vi "CHS_TRAJECTORY_EXECUTE_REL.vi"(6 "Pass_Through_Time":dbl=-1.0 format="%33.4f", 8 "Init":bool, 11 "TrajectoryName":string) -> (1 "Complete":bool, 2 "AtReference":bool, 3 "Chassis Velocity Target SI":T1 {"vOmega" format="%10.3f"; "vY" format="%10.3f"; "vX" format="%10.3f"})   [LabVIEW 2019]
uses:
  CHS_TRAJECTORY_GLOBALS.vi
  <vilib>/Rock Robotics/WPI/ThirdParty/JAS_Junk/TrajLib/Trajectory_Library.lvlib
  <vilib>/Rock Robotics/WPI/ThirdParty/ChoreoLib/ChoreoLib.lvlib
  <vilib>/Rock Robotics/WPI/ThirdParty/JAS_Junk/TrajLib/TypeDef/CHASSIS_SPEEDS.ctl
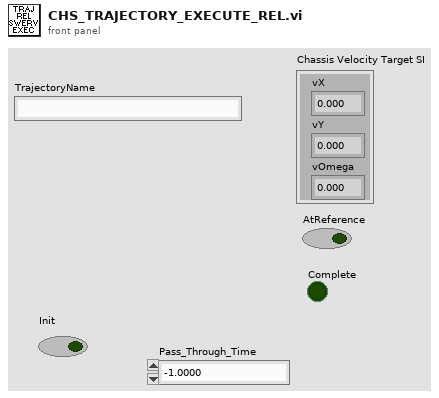
[diagram p1: front panel]
types:
  T1 = typedef "Trajectory_Library.lvlib/CHASSIS_SPEEDS.ctl" = cluster{"vX":dbl, "vY":dbl, "vOmega":dbl}
  T2 = typedef "Trajectory_Library.lvlib/DIFF_DRIVE_KINEMATICS.ctl" = cluster{"TrackWidth_Meters":dbl}
  T3 = typedef "Trajectory_Library.lvlib/SWERVE_DRIVE_MODULE_POSITION.ctl" = cluster{"Distance":dbl, "Angle":T4, "P":bool}
  T4 = typedef "Trajectory_Library.lvlib/ROTATION2D.ctl" = cluster{"VALUE":dbl, "COS":dbl, "SIN":dbl}
  T5 = typedef "Trajectory_Library.lvlib/PID_ADV_LIMITS.ctl" = cluster{"MaxInput":dbl, "MinInput":dbl, "Continuous":bool, "MaxOutput":dbl, "MinOutput":dbl}
  T6 = typedef "Trajectory_Library.lvlib/PID_ADV_TUNING.ctl" = cluster{"Kf":dbl, "Kp":dbl, "Ki":dbl, "Kd":dbl, "MaximumIntegral":dbl, "MinimumIntegral":dbl, "Filter Derivative":bool, "IntegralZone":dbl}
  T7 = typedef "Trajectory_Library.lvlib/POSE2D.ctl" = cluster{"TRANSLATION":T8, "ROTATION":T4}
  T8 = typedef "Trajectory_Library.lvlib/TRANSLATION2D.ctl" = cluster{"X":dbl, "Y":dbl}
  T9 = typedef "ChoreoLib.lvlib/ChoreoSwerveControlConfig.ctl" = cluster{"X_Adv PID Tuning":T6, "X_Adv PID Limits":T5, "Y_Adv PID Tuning":T6, "Y_Adv PID Limits":T5, "Rot_Adv PID Tuning":T6, "Rot_Adv PID Limits":T5, "X Y Pos Tolerance M":dbl, "Rot Tolerance Deg":dbl, "X Y Vel Tolerance M/S":dbl, "Rot Vel Tolerance Deg/S":dbl}
  T10 = cluster{"X Pos Err M":dbl, "X Vel Err M/S":dbl, "Y Pos Err M":dbl, "Y Vel Err M/S":dbl, "Rot Pos Err Deg":dbl, "Rot Vel Err Deg/Sec":dbl}
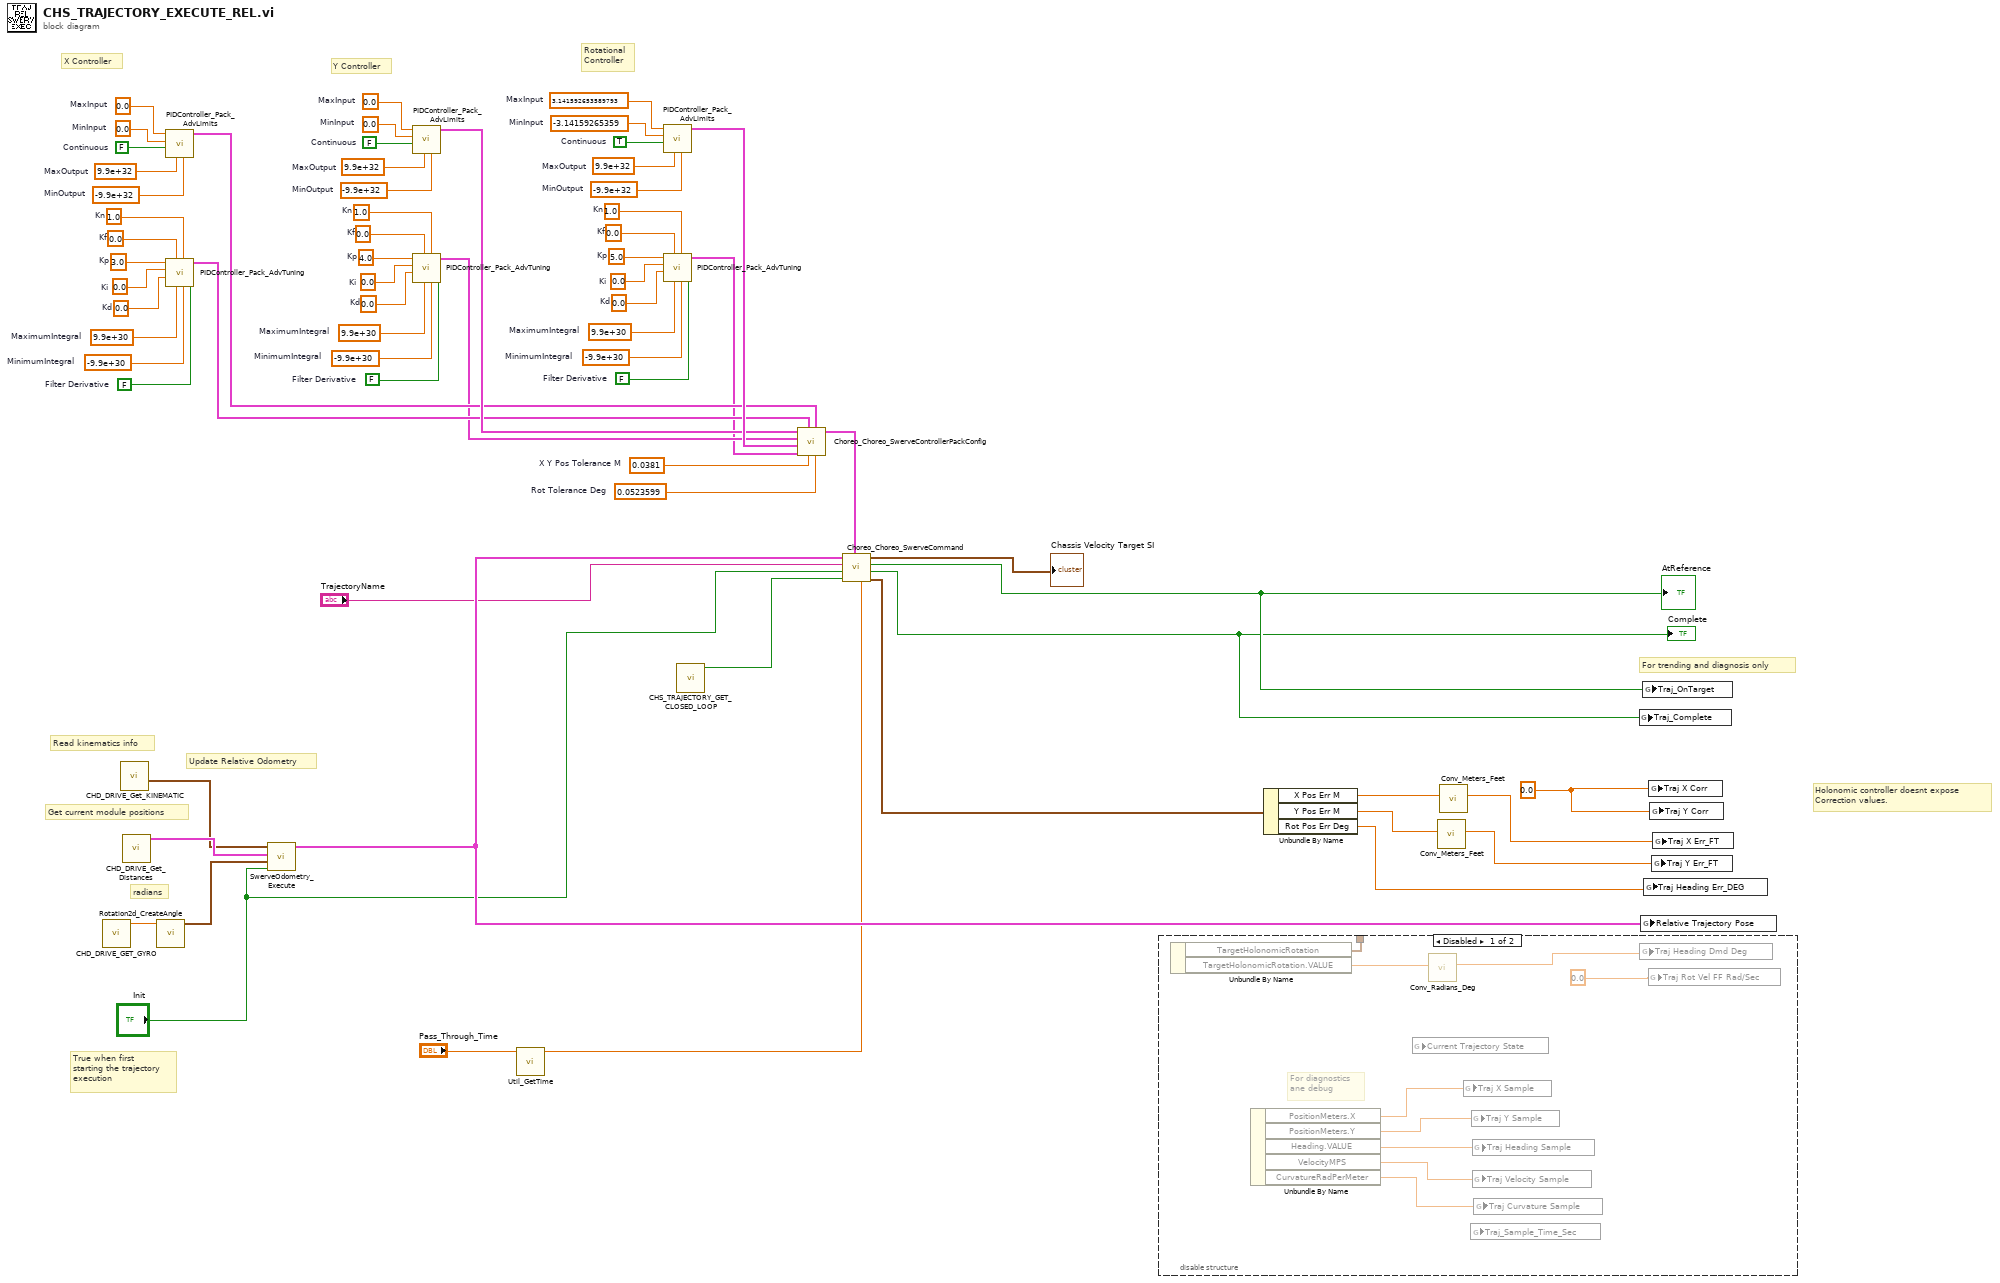
[diagram p0: block diagram]
diagram:
  w8 = 0.0 ("Y Corr")
  w65 = 0.0523599  # Rot Tolerance Deg
  w64 = 0.0381  # X Y Pos Tolerance M
  w45 = 1.0  # Kn
  w46 = 5.0  # Kp
  w47 = 0.0  # Ki
  w48 = 0.0  # Kd
  w49 = 0.0  # Kf
  w50 = 9.9e+30  # MaximumIntegral
  w51 = -9.9e+30  # MinimumIntegral
  w52 = FALSE  # Filter Derivative
  w54 = -3.14159265359  # MinInput
  w55 = TRUE  # Continuous
  w56 = 9.9e+32  # MaxOutput
  w53 = -9.9e+32  # MinOutput
  w57 = 3.141592653589793  # MaxInput
  w32 = 1.0  # Kn
  w33 = 4.0  # Kp
  w34 = 0.0  # Ki
  w35 = 0.0  # Kd
  w36 = 0.0  # Kf
  w37 = 9.9e+30  # MaximumIntegral
  w38 = -9.9e+30  # MinimumIntegral
  w39 = FALSE  # Filter Derivative
  w41 = 0.0  # MinInput
  w42 = FALSE  # Continuous
  w43 = 9.9e+32  # MaxOutput
  w40 = -9.9e+32  # MinOutput
  w44 = 0.0  # MaxInput
  w19 = 1.0  # Kn
  w20 = 3.0  # Kp
  w21 = 0.0  # Ki
  w22 = 0.0  # Kd
  w23 = 0.0  # Kf
  w24 = 9.9e+30  # MaximumIntegral
  w25 = -9.9e+30  # MinimumIntegral
  w26 = FALSE  # Filter Derivative
  w28 = 0.0  # MinInput
  w29 = FALSE  # Continuous
  w30 = 9.9e+32  # MaxOutput
  w27 = -9.9e+32  # MinOutput
  w31 = 0.0  # MaxInput
  # "Rotational\nController"
  # "Y Controller"
  # "X Controller"
  # "Get current module positions"
  # "Update Relative Odometry"
  # "Read kinematics info"
  # "radians"
  # "True when first\nstarting the trajectory\nexecution"
  # "Holonomic controller doesnt expose\nCorrection values."
  # "For trending and diagnosis only"
  n1 = call "CHD_DRIVE_GET_GYRO.vi"() -> ("Gyro Heading Radians"=w9:dbl)  [unwired: 11 in]
  n2 = call "CHD_DRIVE_Get_KINEMATIC.vi"() -> ("out DIFF_DRIVE_KINEMATICS"=w66:T2)  [unwired: 11 in]
  n3 = call "CHD_DRIVE_Get_Distances.vi"() -> ("Swerve Module Positions"=w67:T3[])  [unwired: 11 in]
  n4 = call <vilib>:"Rotation2d_CreateAngle.vi"("Angle"=w9) -> ("ROTATION"=w68:T4)  [unwired: 10 in]
  n5 = call <vilib>:"PIDController_Pack_AdvLimits.vi"("MinOutput"=w27, "MaxOutput"=w30, "Continuous"=w29, "MinInput"=w28, "MaxInput"=w31) -> ("Adv PID Limits"=w61:T5)  [unwired: 6 in]
  n6 = call <vilib>:"PIDController_Pack_AdvTuning.vi"("Filter Derivative"=w26, "MinimumIntegral"=w25, "Kn"=w19, "MaximumIntegral"=w24, "Kf"=w23, "Kd"=w22, "Ki"=w21, "Kp"=w20) -> ("Adv PID Tuning"=w60:T6)  [unwired: 3 in]
  n7 = call <vilib>:"SwerveOdometry_Execute.vi"("Init"="Init", "Rotation"=w68, "Swerve Module Positions"=w67, "SWERVE_DRIVE_KINEMATICS"=w66) -> ("Current Pose"=w17:T7)  [unwired: 5 in, 2 out]
  n8 = call <vilib>:"PIDController_Pack_AdvLimits.vi"("MinOutput"=w40, "MaxOutput"=w43, "Continuous"=w42, "MinInput"=w41, "MaxInput"=w44) -> ("Adv PID Limits"=w62:T5)  [unwired: 6 in]
  n9 = call <vilib>:"PIDController_Pack_AdvTuning.vi"("Filter Derivative"=w39, "MinimumIntegral"=w38, "Kn"=w32, "MaximumIntegral"=w37, "Kf"=w36, "Kd"=w35, "Ki"=w34, "Kp"=w33) -> ("Adv PID Tuning"=w59:T6)  [unwired: 3 in]
  n10 = call <vilib>:"Util_GetTime.vi"("Pass_Through_Time"="Pass_Through_Time") -> ("FPGA_Time_Seconds"=w10:dbl)  [unwired: 8 in, 2 out]
  n11 = call <vilib>:"PIDController_Pack_AdvLimits.vi"("MinOutput"=w53, "MaxOutput"=w56, "Continuous"=w55, "MinInput"=w54, "MaxInput"=w57) -> ("Adv PID Limits"=w63:T5)  [unwired: 6 in]
  n12 = call <vilib>:"PIDController_Pack_AdvTuning.vi"("Filter Derivative"=w52, "MinimumIntegral"=w51, "Kn"=w45, "MaximumIntegral"=w50, "Kf"=w49, "Kd"=w48, "Ki"=w47, "Kp"=w46) -> ("Adv PID Tuning"=w58:T6)  [unwired: 3 in]
  n13 = call "CHS_TRAJECTORY_GET_CLOSED_LOOP.vi"() -> ("AUTO_CLOSED_LOOP"=w13:bool)  [unwired: 11 in]
  n14 = call <vilib>:"Choreo_Choreo_SwerveControllerPackConfig.vi"("Rot Tolerance Deg"=w65, "X_Adv PID Limits"=w61, "X Y Pos Tolerance M"=w64, "X_Adv PID Tuning"=w60, "Rot_Adv PID Tuning"=w58, "Rot_Adv PID Limits"=w63, "Y_Adv PID Tuning"=w59, "Y_Adv PID Limits"=w62) -> ("ChoreoSwerveControlConfig"=w18:T9)  [unwired: 3 in]
  n15 = call <vilib>:"Choreo_Choreo_SwerveCommand.vi"("Pass_Through_Time"=w10, "ChoreoSwerveControlConfig"=w18, "Auto"=w13, "Initialize"="Init", "TrajectoryName"="TrajectoryName", "Current Position"=w17) -> ("Ctrl Info"=w5:T10, "Complete"=w14:bool, "On Target"=w15:bool, "Chassis Speed Dmd"=→"Chassis Velocity Target SI":T1)  [unwired: 2 in]
  "AtReference" <- w15
  "Complete" <- w14
  n16 = disable-structure shown="Disabled" {
    disable-tunnel: [w69 _] -> _
    frame Disabled {
      # "For diagnostics\nane debug"
      n17 = Unbundle By Name() -> ("TargetHolonomicRotation"=w69:T4, "TargetHolonomicRotation.VALUE"=w71:dbl)  [unwired: 1 in]
      n18 = Unbundle By Name() -> ("PositionMeters.X"=w77:dbl, "PositionMeters.Y"=w76:dbl, "Heading.VALUE"=w75:dbl, "VelocityMPS"=w74:dbl, "CurvatureRadPerMeter"=w73:dbl)  [unwired: 1 in]
      n19 = global read "CHS_TRAJECTORY_GLOBALS.vi" "Current Trajectory State"() -> ()  [unwired: 1 in]
      n20 = call <vilib>:"Conv_Radians_Deg.vi"("Radians"=w71) -> ("Degrees"=w70:dbl)  [unwired: 10 in]
      n21 = global write "CHS_TRAJECTORY_GLOBALS.vi" "Traj X Sample"(w77) -> ()
      n22 = global read "CHS_TRAJECTORY_GLOBALS.vi" "Traj_Sample_Time_Sec"() -> ()  [unwired: 1 in]
      n23 = global write "CHS_TRAJECTORY_GLOBALS.vi" "Traj Y Sample"(w76) -> ()
      n24 = global write "CHS_TRAJECTORY_GLOBALS.vi" "Traj Heading Sample"(w75) -> ()
      n25 = global write "CHS_TRAJECTORY_GLOBALS.vi" "Traj Velocity Sample"(w74) -> ()
      n26 = global write "CHS_TRAJECTORY_GLOBALS.vi" "Traj Curvature Sample"(w73) -> ()
      n27 = global write "CHS_TRAJECTORY_GLOBALS.vi" "Traj Heading Dmd Deg"(w70) -> ()
      n28 = global write "CHS_TRAJECTORY_GLOBALS.vi" "Traj Rot Vel FF Rad/Sec"(0.0 ("Traj Heading Dmd Deg")) -> ()
    }
    frame Enabled {
    }
  }
  n29 = Unbundle By Name(w5) -> ("X Pos Err M"=w7:dbl, "Y Pos Err M"=w6:dbl, "Rot Pos Err Deg"=w2:dbl)
  n30 = call <vilib>:"Conv_Meters_Feet.vi"("Meters"=w6) -> ("Feet"=w3:dbl)  [unwired: 10 in]
  n31 = call <vilib>:"Conv_Meters_Feet.vi"("Meters"=w7) -> ("Feet"=w4:dbl)  [unwired: 10 in]
  n32 = global write "CHS_TRAJECTORY_GLOBALS.vi" "Traj_Complete"(w14) -> ()
  n33 = global write "CHS_TRAJECTORY_GLOBALS.vi" "Relative Trajectory Pose"(w17) -> ()
  n34 = global write "CHS_TRAJECTORY_GLOBALS.vi" "Traj_OnTarget"(w15) -> ()
  n35 = global write "CHS_TRAJECTORY_GLOBALS.vi" "Traj Heading Err_DEG"(w2) -> ()
  n36 = global write "CHS_TRAJECTORY_GLOBALS.vi" "Traj X Corr"(w8) -> ()
  n37 = global write "CHS_TRAJECTORY_GLOBALS.vi" "Traj Y Corr"(w8) -> ()
  n38 = global write "CHS_TRAJECTORY_GLOBALS.vi" "Traj Y Err_FT"(w3) -> ()
  n39 = global write "CHS_TRAJECTORY_GLOBALS.vi" "Traj X Err_FT"(w4) -> ()
